vi "Destroy User Events.vi"(11 "UI Template in":refnum<class "Network Management UI.lvclass">) -> (3 "UI Template out":refnum<class "Network Management UI.lvclass">)   [LabVIEW 2020, in "Network Management UI.lvlib" / "Network Management UI.lvclass"]
uses:
  Network Management UI.lvclass
  Network Management UI.lvclass/Network Management UI.ctl
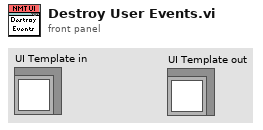
[diagram p1: front panel]
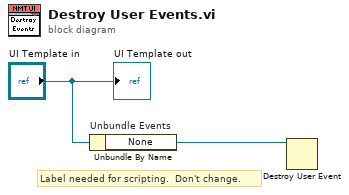
[diagram p0: block diagram]
diagram:
  # "Label needed for scripting.  Don't change."
  n1 = Unbundle By Name "Unbundle Events"("UI Template in") -> ("None"=w2:refnum<user-event>)
  n2 = Destroy User Event(user event=w2) -> ()  [unwired: 1 in, 1 out]
  "UI Template out" <- "UI Template in"
